vi "Error Query.vi"(8 "error in (no error)":errorcluster, 10 "parseError? (true)":bool=TRUE, 11 "VISA resource name":refnum<visa-resource-name>) -> (0 "error out":errorcluster, 1 "Code":i32, 2 "AnswerString (output)":string, 3 "VISA resource name out":refnum<visa-resource-name>)   [LabVIEW 2018, in "JULABO DeviceDriver.lvlib"]
doc: "Queries the instrument for any errors in the instrument's error queue. It will continue to read errors until all errors have been read from the instrument. Any errors will be returned in the Error Out cluster.\n\nNote:\nThis VI is called automatically by most driver VIs so it is not usually necessary to call this in an application."
uses:
  JULABO DeviceDriver.lvlib
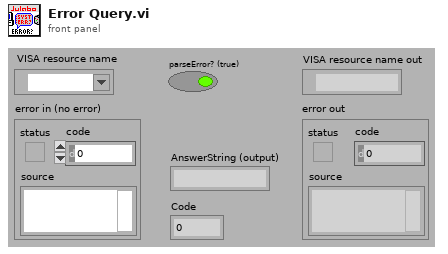
[diagram p1: front panel]
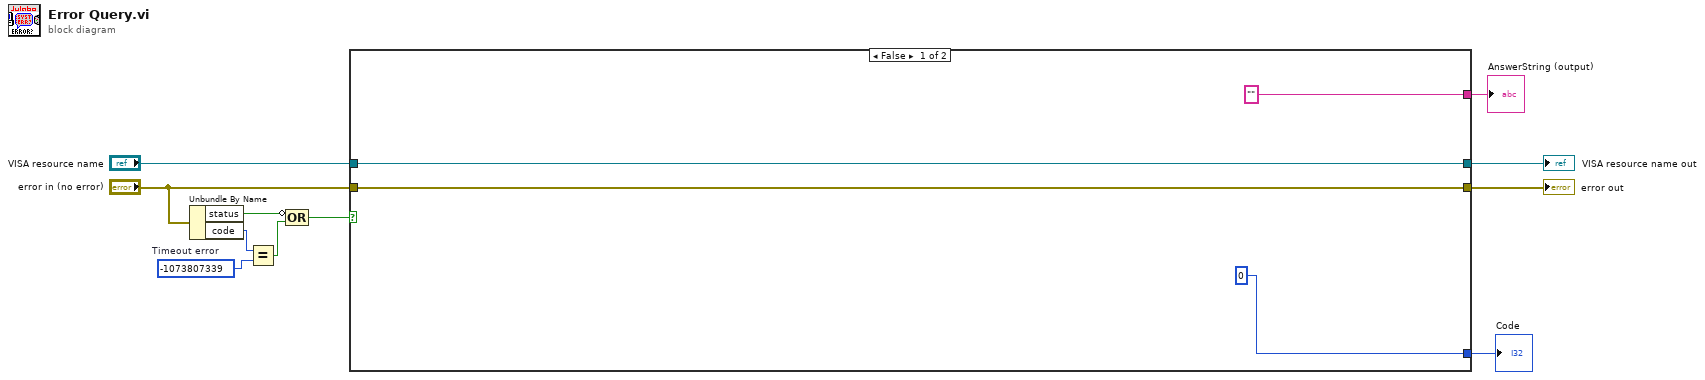
[diagram p0: block diagram]
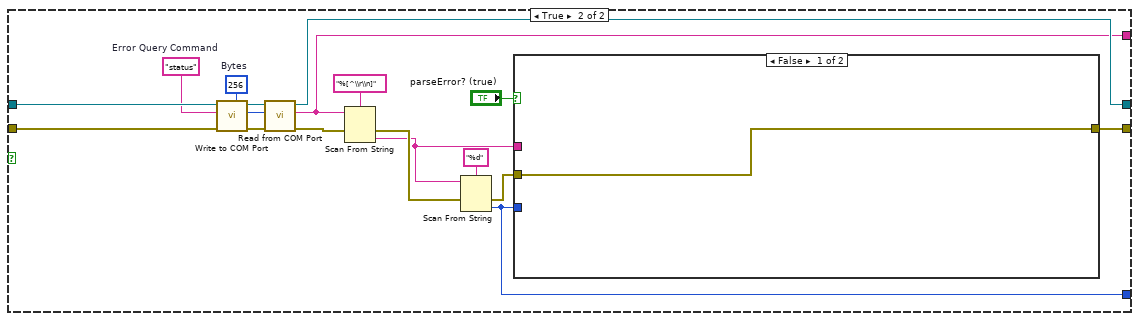
[diagram p2: hidden frame]
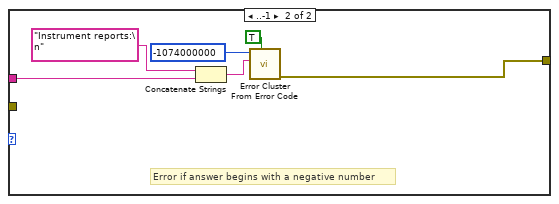
[diagram p4: hidden frame]
diagram:
  w4 = -1073807339  # Timeout error
  n1 = Unbundle By Name("error in (no error)") -> ("status"=w3:bool, "code"=w6:i32)
  n2 = Equal?(x=w6, y=w4) -> (x = y?=w5:bool)
  n3 = Compound Arithmetic op=OR(invert w3, w5) -> (w2:bool)
  n4 = case shown="False" w2 {
    tunnel: [w15 w20] -> w11
    tunnel: "VISA resource name" -> [w15 w32]
    tunnel: [w12 w23] -> w9
    tunnel: ["" ("String (output)") w19] -> w8
    tunnel: [0 w18] -> w7
    tunnel: "error in (no error)" -> [w12 w17]
    frame False {
    }
    frame True {
      w30 = u32 256  # Bytes
      w28 = "status"  # Error Query Command
      n5 = call "Write to COM Port.vi"("error in"=w17, "Command (input)"=w28, "VISA resource name in"=w32) -> ("error out"=w29:errorcluster, "VISA resource name out"=w31:refnum<visa-resource-name>)  [unwired: 7 in]
      n6 = call "Read from COM Port.vi"("error in"=w29, "Byte to Read (-1:All)"=w30, "VISA resource name in"=w31) -> ("error out"=w25:errorcluster, "String (output)"=w19:string, "VISA resource name out"=w20:refnum<visa-resource-name>)  [unwired: 5 in, 1 out]
      n7 = Scan From String(format string="%[^\\r\\n]", input string=w19, error in=w25) -> (error out=w24:errorcluster, output 1=w16:string)  [unwired: 2 in, 2 out]
      n8 = Scan From String(format string="%d", input string=w16, error in=w24) -> (error out=w22:errorcluster, output 1=w18:i32)  [unwired: 2 in, 2 out]
      n9 = case shown="False" "parseError? (true)" {
        tunnel: w18 -> [_ w37]
        tunnel: w16 -> [_ w36]
        tunnel: [w33 w35] -> w23
        tunnel: w22 -> [w33 w34]
        frame False {
        }
        frame True {
          n10 = case shown="Default" w37 {
            tunnel: w36 -> [_ w40]
            tunnel: [w38 w39] -> w35
            tunnel: w34 -> [w38 _]
            frame Default {
            }
            frame ..-1 {
              # "Error if answer begins with a negative number"
              # "-08 INVALID COMMAND\n-09 COMMAND NOT ALLOWED IN CURRENT OPERATING MODE"
              n11 = Concatenate Strings("Instrument reports:\n" ("Source"), w40) -> (w44:string)
              n12 = call <vilib>:"Error Cluster From Error Code.vi"("show call chain? (False)"=TRUE, "error message (\"\")"=w44, "error code (0)"=-1074000000 ("Code")) -> ("error out"=w39:errorcluster)  [unwired: 6 in]
            }
          }
        }
      }
    }
  }
  "VISA resource name out" <- w11
  "error out" <- w9
  "AnswerString (output)" <- w8
  "Code" <- w7
